vi "警示对话框.vi"(5 "副标题颜色":u32(colorbox), 7 "主标题颜色":u32(colorbox), 10 "副标题":string, 11 "主标题":string) -> (2 "check":bool)   [LabVIEW 2016, in "斯坦道总氮.lvlib"]
panel:
  in  "取消":bool
  in  "确认":bool
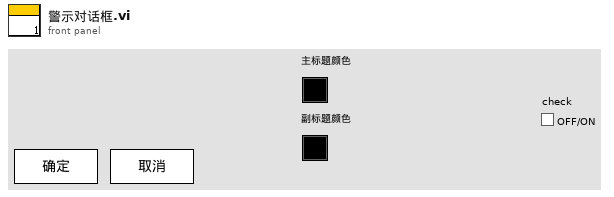
[diagram p1: front panel]
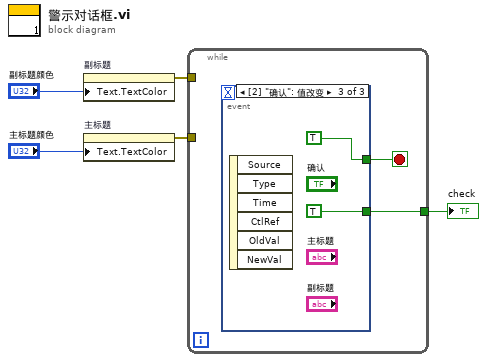
[diagram p0: block diagram]
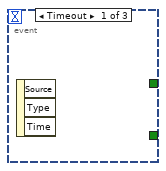
[diagram p2: hidden frame]
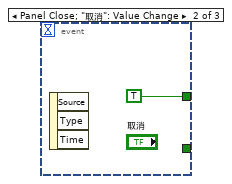
[diagram p3: hidden frame]
diagram:
  n1 = property on="副标题" class="Str"("Text.TextColor"="副标题颜色") -> (error out=w3:errorcluster)  [unwired: 2 in, 1 out]
  n2 = property on="主标题" class="Str"("Text.TextColor"="主标题颜色") -> (error out=w2:errorcluster)  [unwired: 2 in, 1 out]
  n3 = while {
    tunnel: w3 -> [_]
    tunnel: w2 -> [_]
    tunnel: [w6] -> w1
    stop <- w7 stop-if-true
    n4 = event shown="[2] \"确认\": 值改变" {
      selector: _ -> [_ _ _]
      dyn-events: _ -> [_ _ _]
      timeout: _ -> [_ _ _]
      tunnel: [_ TRUE TRUE] -> w7
      tunnel: [_ _ TRUE] -> w6
      event Timeout {
        n5 = event-data() -> ()  [unwired: 1 in, 3 out]
      }
      event Panel Close; "取消": Value Change {
        n6 = event-data() -> ()  [unwired: 1 in, 3 out]
      }
      event "确认": Value Change {
        n7 = event-data() -> ()  [unwired: 1 in, 6 out]
      }
    }
  }
  "check" <- w1
